vi "fit01.vi"(2 "input":T1) -> (0 "fitness":dbl=1.2)   [LabVIEW 2013]
uses:
  <vilib>/Analysis/Matrix/Datatypes/RealMatrix.ctl
  <vilib>/Analysis/baseanly.llb/Mean (DBL).vi
  <vilib>/Analysis/Matrix/Numeric/Conversions/Matrix To Array - RM.vi
  <vilib>/Analysis/NI_AALBase.lvlib
  <vilib>/Analysis/Matrix/NI_Matrix.lvlib
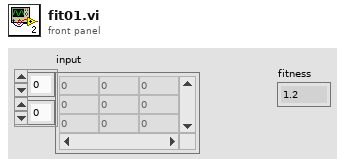
[diagram p1: front panel]
types:
  T1 = typedef "NI_Matrix.lvlib/RealMatrix.ctl" = dbl[][]
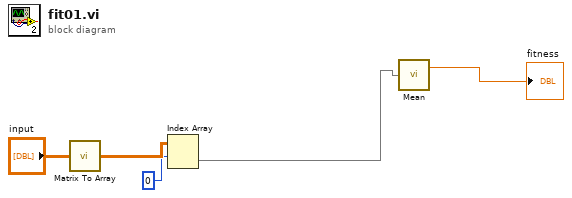
[diagram p0: block diagram]
diagram:
  n1 = call-poly <vilib>:"Matrix To Array.vi"("Real Matrix"="input") -> ("Real 2D Array"=w3:dbl[][])
  n2 = Index Array(array=w3, index (row)=0) -> (element=w1:dbl[])  [unwired: 1 in]
  n3 = call-poly <vilib>:"Mean.vi"("X"=w1) -> ("mean"=→"fitness":dbl)  [unwired: 1 out]
